vi "Test Load MP3.vi"(8 "error in (no error)":errorcluster) -> (0 "error out":errorcluster, 3 "Pass?":bool)   [LabVIEW 2020]
uses:
  558d703f-9b78-4752-b6ca-da8df52f0aac.vi
  <vilib>/sound2/lvsound2.llb/Sound File Read Open.vi
  <vilib>/sound2/lvsound2.llb/Sound File Info (refnum).vi
  <vilib>/sound2/lvsound2.llb/Sound File Read (I16).vi
  G-Audio/G-Audio.lvlib
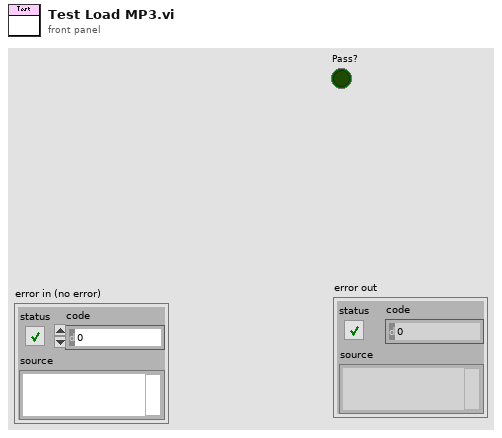
[diagram p1: front panel]
types:
  T1 = typedef "Sound File Refnum.ctl" = refnum<file>
  T2 = typedef "Sound Data Format.ctl" = cluster{"sample rate (S/s)":dbl, "number of channels":i32, "bits per sample":i32}
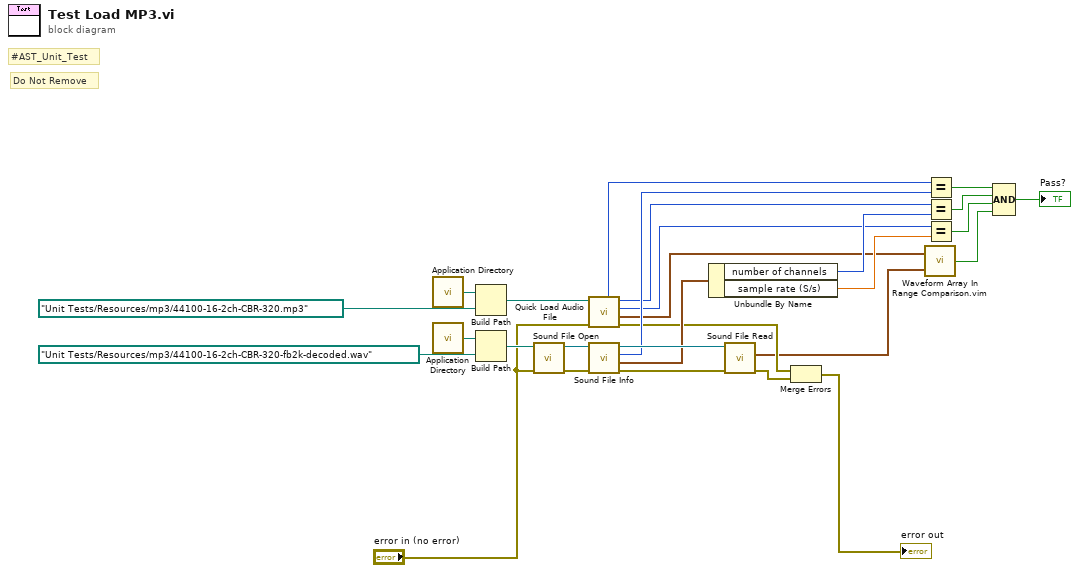
[diagram p0: block diagram]
diagram:
  # "Do Not Remove"
  # "#AST_Unit_Test"
  n1 = call <vilib>:"Application Directory.vi"() -> ("Application Directory"=w3:path)
  n2 = call <vilib>:"Application Directory.vi"() -> ("Application Directory"=w28:path)
  n3 = Build Path(base path=w3, name or relative path=path "Unit Tests/Resources/mp3/44100-16-2ch-CBR-320.mp3" ("Path")) -> (appended path=w1:path)
  n4 = Build Path(base path=w28, name or relative path=path "Unit Tests/Resources/mp3/44100-16-2ch-CBR-320-fb2k-decoded.wav" ("Path")) -> (appended path=w27:path)
  n5 = call-poly <vilib>:"Sound File Open.vi"("error in (no error)"="error in (no error)", "path"=w27) -> ("error out"=w13:errorcluster, "sound file refnum"=w25:T1)  [unwired: 8 in]
  n6 = call "Quick Load Audio File.vi"("error in (no error)"="error in (no error)", "Path"=w1) -> ("error out"=w10:errorcluster, "data"=w5:waveform(i16)[], "Sample Rate (Hz)"=w16:u32, "Channels"=w18:u32, "Length (Samples)"=w21:u64)  [unwired: 5 in]
  n7 = call-poly <vilib>:"Sound File Info.vi"("error in (no error)"=w13, "sound file refnum"=w25) -> ("error out"=w12:errorcluster, "sound format"=w19:T2, "total number of samples/ch"=w20:u32, "sound file refnum out"=w24:T1)  [unwired: 6 in]
  n8 = Unbundle By Name(w19) -> ("number of channels"=w17:i32, "sample rate (S/s)"=w7:dbl)
  n9 = call-poly <vilib>:"Sound File Read.vi"("error in (no error)"=w12, "sound file refnum"=w24) -> ("error out"=w9:errorcluster, "data"=w6:waveform(i16)[])  [unwired: 5 in, 3 out]
  n10 = Merge Errors(w10, w9) -> (→"error out":errorcluster)
  n11 = call "Waveform Array In Range Comparison.vim"("Expected Value"=w6, "Resulting Value"=w5) -> ("Comparison Result"=w4:bool)
  n12 = Equal?(x=w21, y=w20) -> (x = y?=w23:bool)
  n13 = Equal?(x=w18, y=w17) -> (x = y?=w15:bool)
  n14 = Equal?(x=w16, y=w7) -> (x = y?=w14:bool)
  n15 = Compound Arithmetic op=AND(w23, w15, w14, w4) -> (→"Pass?":bool)
